vi "BRig_RT__Case_Exp__State_ENL__v3.vi"(0 "input_dataCurrent":u16[](array[numeric]), 1 "input_dataTrial":u16[][](array[numeric]), 3 "input_ENL2":bool, 5 "input_arrTrig":bool[](array[boolean]), 6 "input_state":T1, 8 "I_lick":bool) -> (7 "output_l2_laserOn":bool, 9 "output_l2_laserEvent":bool, 11 "output_l1_laserOn":bool, 12 "output_state":T1, 13 "output_l1_laserEvent":bool, 14 "output_dataCurrent":u16[](array[numeric]), 15 "output_dataTrial":u16[][](array[numeric]))   [LabVIEW 2014]
uses:
  myRIO_BRig_RT__Case_Exp_stateList.ctl
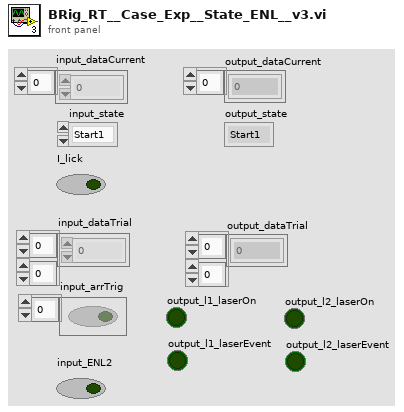
[diagram p1: front panel]
types:
  T1 = typedef "myRIO_BRig_RT__Case_Exp_stateList.ctl" = enum16{"Start1", "Start2", "Start3", "saveSettings1", "saveSettings2", "saveSettings3", "saveSettings4", "saveSettings_LC_ENL_l1", "saveSettings_LC_ENL_l2", "saveSettings_LC_Cue_l1", "saveSettings_LC_Cue_l2", "saveSettings6_LC_l1_Other", "SaveSettings6_LC_l2_Other", "setSettings_Audio", "setSettings_Laser", "initBlock_pre", "initBlock", "initBlock2", "initBlock_post", "initTrial_pre", "initTrial", "initTrial2", "initTrial3", "initTrial4", "initTrial_LC_ENL1", "initTrial_LC_Cue1", "initTrial_LC_Cue1_2", "initTrial_LC_Sel", "initTrial_post", "ENL1_pre", "ENL1", "ENL1_post", "ENL1Penalty_pre", "ENL1Penalty", "ENL2_pre", "ENL2", "ENL2Penalty_pre", "ENL2Penalty", "Cue1_pre", "Cue1", "Cue1_post", "Cue1Penalty_pre", "Cue1Penalty", "Cue2_pre", "Cue2", "Cue2Penalty_pre", "Cue2Penalty", "Selection_pre", "Selection", "Select_post", "SelectReward_pre", "SelectReward", "SelectRewardPost_pre", "SelectRewardPost", "SelectWrong_pre", "SelectWrong", "SelectWrong_post", "SelectTimeout_pre", "SelectTimeout", "SelectTimeout_post", "endTrial_pre", "endTrial1", "endTrial2", "endTrial3", "endTrial_post", "endBlock_pre", "endBlock", "endBlock_post", "endExp", "commConnect", "commUpload_pre", "commUpload_dataBlock", "commUpload_dataCurrent", "commUpload_dataExp", "commUpload_dataLC", "commUpload_dataTrial", "commUpload_post", "saveData_pre", "saveData_dataBlock", "saveData_dataCurrent", "saveData_dataExp", "saveData_dataLC", "saveData_dataTrial", "saveData_post", "empty_endBlock1", "empty_endBlock2", "empty_endTrial1", "empty_endTrial2", "empty_endTrial3", "empty_endTrial4", "empty_endTrial5", "dummyState", "dummyState_endBlock", "FreeReward_pre", "FreeReward", "FreeRewardPost_pre", "FreeRewardPost"}
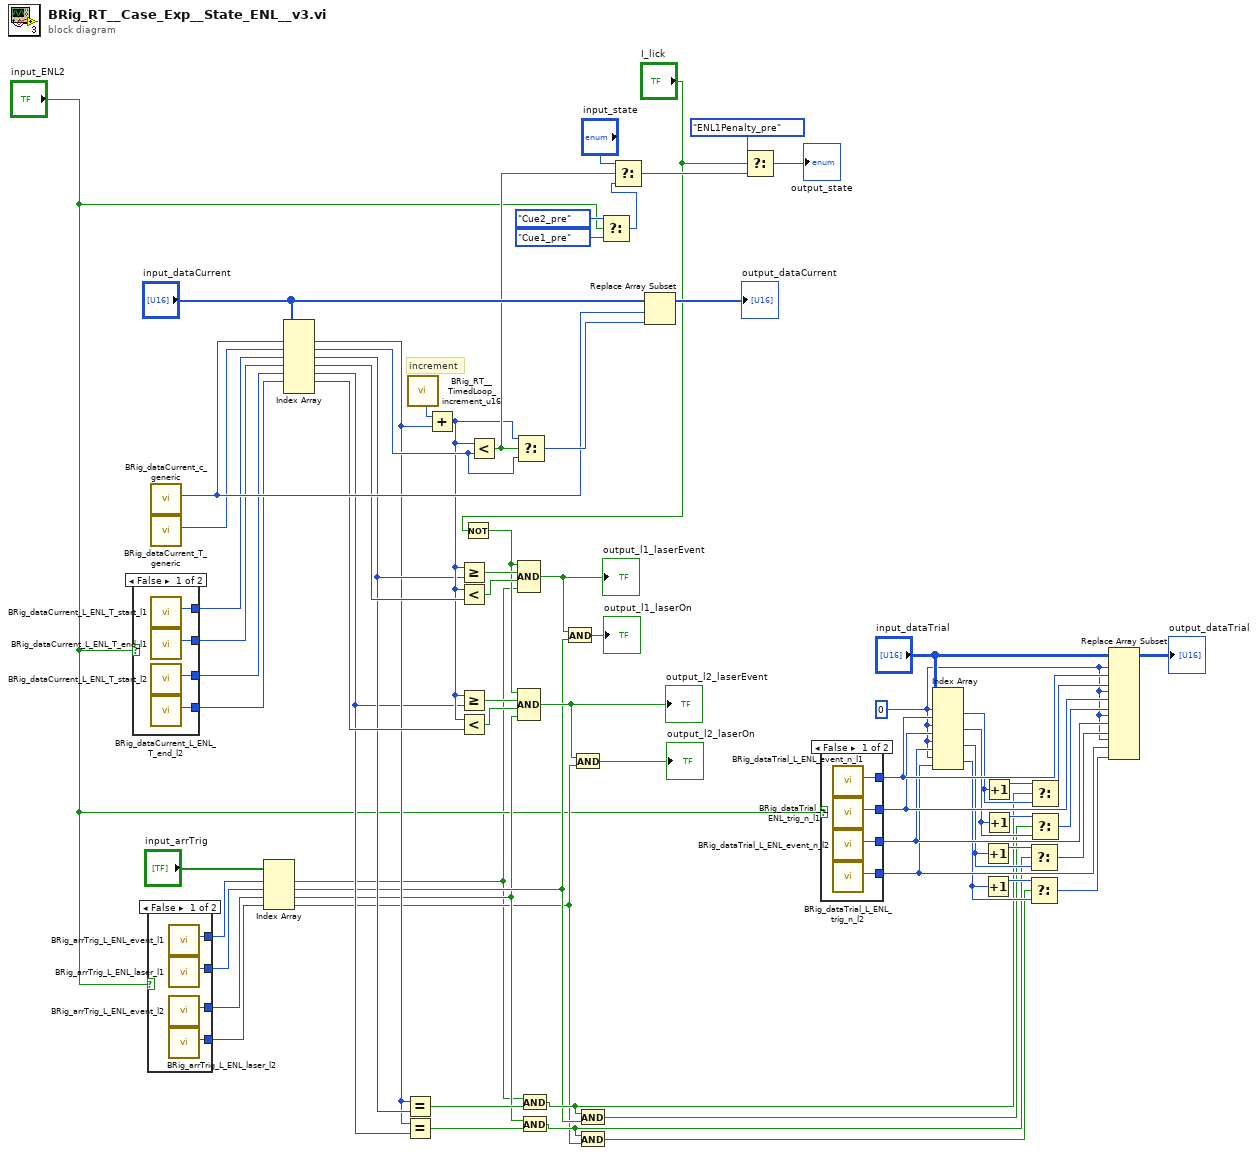
[diagram p0: block diagram]
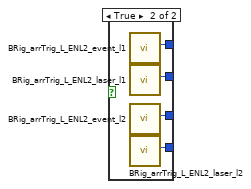
[diagram p2: hidden frame]
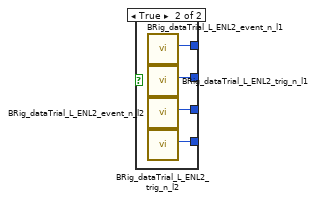
[diagram p3: hidden frame]
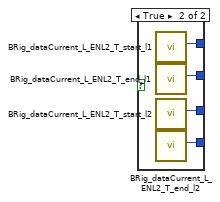
[diagram p4: hidden frame]
diagram:
  w13 = 0
  # "increment"
  n1 = case shown="False" "input_ENL2" {
    tunnel: [w74 w78] -> w49
    tunnel: [w73 w77] -> w48
    tunnel: [w72 w76] -> w47
    tunnel: [w71 w75] -> w46
    frame False {
      n2 = call "BRig_dataCurrent_L_ENL_T_start_l1.vi"() -> ("output_L_ENL_T_start_l1"=w74:i32)  [unwired: 11 in]
      n3 = call "BRig_dataCurrent_L_ENL_T_end_l1.vi"() -> ("output_L_ENL_T_end_l1"=w73:i32)  [unwired: 11 in]
      n4 = call "BRig_dataCurrent_L_ENL_T_start_l2.vi"() -> ("output_L_T_ENL1_start_l2"=w72:i32)  [unwired: 11 in]
      n5 = call "BRig_dataCurrent_L_ENL_T_end_l2.vi"() -> ("output_L_ENL_T_end_l2"=w71:i32)  [unwired: 11 in]
    }
    frame True {
      n6 = call "BRig_dataCurrent_L_ENL2_T_start_l1.vi"() -> ("output_L_ENL2_T_start_l1"=w78:i32)  [unwired: 11 in]
      n7 = call "BRig_dataCurrent_L_ENL2_T_end_l1.vi"() -> ("output_L_ENL2_T_end_l1"=w77:i32)  [unwired: 11 in]
      n8 = call "BRig_dataCurrent_L_ENL2_T_start_l2.vi"() -> ("output_L_T_ENL2_start_l2"=w76:i32)  [unwired: 11 in]
      n9 = call "BRig_dataCurrent_L_ENL2_T_end_l2.vi"() -> ("output_L_ENL2_T_end_l2"=w75:i32)  [unwired: 11 in]
    }
  }
  n10 = case shown="False" "input_ENL2" {
    tunnel: [w82 w86] -> w40
    tunnel: [w81 w85] -> w39
    tunnel: [w80 w84] -> w38
    tunnel: [w79 w83] -> w37
    frame False {
      n11 = call "BRig_arrTrig_L_ENL_event_l1.vi"() -> ("output_L_ENL_event_l1"=w82:i32)  [unwired: 11 in]
      n12 = call "BRig_arrTrig_L_ENL_laser_l1.vi"() -> ("output_L_ENL_laserTrig_l1"=w81:i32)  [unwired: 11 in]
      n13 = call "BRig_arrTrig_L_ENL_event_l2.vi"() -> ("output_L_ENL_event_l2"=w80:i32)  [unwired: 11 in]
      n14 = call "BRig_arrTrig_L_ENL_laser_l2.vi"() -> ("output_L_ENL_laserTrig_l2"=w79:i32)  [unwired: 11 in]
    }
    frame True {
      n15 = call "BRig_arrTrig_L_ENL2_event_l1.vi"() -> ("output_L_ENL2_event_l1"=w86:i32)  [unwired: 11 in]
      n16 = call "BRig_arrTrig_L_ENL2_laser_l1.vi"() -> ("output_L_ENL2_laserTrig_l1"=w85:i32)  [unwired: 11 in]
      n17 = call "BRig_arrTrig_L_ENL2_event_l2.vi"() -> ("output_L_ENL2_event_l2"=w84:i32)  [unwired: 11 in]
      n18 = call "BRig_arrTrig_L_ENL2_laser_l2.vi"() -> ("output_L_ENL2_laserTrig_l2"=w83:i32)  [unwired: 11 in]
    }
  }
  n19 = call "BRig_dataCurrent_c_generic.vi"() -> ("output_count_generic"=w52:i32)  [unwired: 11 in]
  n20 = call "BRig_dataCurrent_T_generic.vi"() -> ("output_T_generic"=w51:i32)  [unwired: 11 in]
  n21 = Index Array(array="input_arrTrig", index #1=w40, index #2=w39, index #3=w38, index #4=w37) -> (element #1=w1:bool, element #2=w11:bool, element #3=w7:bool, element #4=w6:bool)
  n22 = Index Array(array="input_dataCurrent", index #1=w52, index #2=w51, index #3=w49, index #4=w48, index #5=w47, index #6=w46) -> (element #1=w35:u16, element #2=w50:u16, element #3=w36:u16, element #4=w44:u16, element #5=w34:u16, element #6=w41:u16)  [unwired: 1 in, 1 out]
  n23 = Equal?(x=w35, y=w36) -> (x = y?=w10:bool)
  n24 = Equal?(x=w35, y=w34) -> (x = y?=w9:bool)
  n25 = call "BRig_RT__TimedLoop_increment_u16.vi"() -> ("output_increment__u16"=w65:u16)  [unwired: 11 in]
  n26 = Add(x=w65, y=w35) -> (x+y=w42:u16)
  n27 = Greater Or Equal?(x=w42, y=w36) -> (x >= y?=w63:bool)
  n28 = Less?(x=w42, y=w44) -> (x < y?=w64:bool)
  n29 = Greater Or Equal?(x=w42, y=w34) -> (x >= y?=w56:bool)
  n30 = Less?(x=w42, y=w41) -> (x < y?=w55:bool)
  n31 = Not(x="I_lick") -> (.not. x?=w43:bool)
  n32 = Less?(x=w42, y=w50) -> (x < y?=w67:bool)
  n33 = Select(t=w42, s=w67, f=w50) -> (s? t:f=w68:u16)
  n34 = Compound Arithmetic op=AND(w43, w63, w64, w1) -> (w58:bool)
  "output_l1_laserEvent" <- w58
  n35 = Compound Arithmetic op=AND(w43, w56, w55, w7) -> (w54:bool)
  "output_l2_laserEvent" <- w54
  n36 = And(x=w1, y=w10) -> (x .and. y?=w12:bool)
  n37 = And(x=w7, y=w9) -> (x .and. y?=w8:bool)
  n38 = And(x=w58, y=w11) -> (x .and. y?=→"output_l1_laserOn":bool)
  n39 = And(x=w54, y=w6) -> (x .and. y?=→"output_l2_laserOn":bool)
  n40 = And(x=w12, y=w11) -> (x .and. y?=w20:bool)
  n41 = And(x=w8, y=w6) -> (x .and. y?=w19:bool)
  n42 = Select(t=myRIO_BRig_RT__Case_Exp_stateList."Cue2_pre" ("Enum"), s="input_ENL2", f=myRIO_BRig_RT__Case_Exp_stateList."Cue1_pre" ("Enum")) -> (s? t:f=w4:T1)
  n43 = Select(t="input_state", s=w67, f=w4) -> (s? t:f=w66:T1)
  n44 = Replace Array Subset(array="input_dataCurrent", new element=w68, index=w52) -> (→"output_dataCurrent":u16[])
  n45 = Select(t=myRIO_BRig_RT__Case_Exp_stateList."ENL1Penalty_pre" ("Enum"), s="I_lick", f=w66) -> (s? t:f=→"output_state":T1)
  n46 = case shown="False" "input_ENL2" {
    tunnel: [w90 w94] -> w32
    tunnel: [w89 w93] -> w31
    tunnel: [w88 w92] -> w30
    tunnel: [w87 w91] -> w29
    frame False {
      n47 = call "BRig_dataTrial_L_ENL_event_n_l1.vi"() -> ("output_L_ENL_event_n_l1"=w90:i32)  [unwired: 11 in]
      n48 = call "BRig_dataTrial_L_ENL_trig_n_l1.vi"() -> ("output_L_ENL_trig_n_l1"=w89:i32)  [unwired: 11 in]
      n49 = call "BRig_dataTrial_L_ENL_event_n_l2.vi"() -> ("output_L_ENL_event_n_l2"=w88:i32)  [unwired: 11 in]
      n50 = call "BRig_dataTrial_L_ENL_trig_n_l2.vi"() -> ("output_L_ENL_trig_n_l2"=w87:i32)  [unwired: 11 in]
    }
    frame True {
      n51 = call "BRig_dataTrial_L_ENL2_event_n_l1.vi"() -> ("output_L_ENL2_event_n_l1"=w94:i32)  [unwired: 11 in]
      n52 = call "BRig_dataTrial_L_ENL2_trig_n_l1.vi"() -> ("output_L_ENL2_trig_n_l1"=w93:i32)  [unwired: 11 in]
      n53 = call "BRig_dataTrial_L_ENL2_event_n_l2.vi"() -> ("output_L_ENL2_event_n_l2"=w92:i32)  [unwired: 11 in]
      n54 = call "BRig_dataTrial_L_ENL2_trig_n_l2.vi"() -> ("output_L_ENL2_trig_n_l2"=w91:i32)  [unwired: 11 in]
    }
  }
  n55 = Index Array(array="input_dataTrial", index (row) #1=w13, index (col) #1=w32, index (row) #2=w13, index (col) #2=w31, index (row) #3=w13, index (col) #3=w30, index (row) #4=w13, index (col) #4=w29) -> (element #1=w27:u16, element #2=w23:u16, element #3=w22:u16, element #4=w21:u16)
  n56 = Increment(x=w22) -> (x+1=w25:u16)
  n57 = Increment(x=w21) -> (x+1=w24:u16)
  n58 = Increment(x=w27) -> (x+1=w28:u16)
  n59 = Increment(x=w23) -> (x+1=w26:u16)
  n60 = Select(t=w25, s=w8, f=w22) -> (s? t:f=w16:u16)
  n61 = Select(t=w24, s=w19, f=w21) -> (s? t:f=w15:u16)
  n62 = Select(t=w28, s=w12, f=w27) -> (s? t:f=w18:u16)
  n63 = Select(t=w26, s=w20, f=w23) -> (s? t:f=w17:u16)
  n64 = Replace Array Subset(array="input_dataTrial", new element #1=w18, index (row) #1=w13, index (col) #1=w32, new element #2=w17, index (row) #2=w13, index (col) #2=w31, new element #3=w16, index (row) #3=w13, index (col) #3=w30, new element #4=w15, index (row) #4=w13, index (col) #4=w29) -> (→"output_dataTrial":u16[][])
